vi "weightedPIDs_Controller_CHN.vi"(0 "PID Array":T4(array[cluster])=[{"proportional gain (Kc)"=0.1, "integral time (Ti, min)"=0.1, "derivative time (Td, min)"=0.0}, {"proportional gain (Kc)"=0.1, "integral time (Ti, min)"=0.1, "derivative time (Td, min)"=0.0}, {"proportional gain (Kc)"=0.1, "integral time (Ti, min)"=0.0, "derivative time (Td, min)"=0.0}, {"proportional gain (Kc)"=0.1, "integral time (Ti, min)"=0.0, "derivative time (Td, min)"=0.0}, {"proportional gain (Kc)"=0.37, "integral time (Ti, min)"=0.16, "derivative time (Td, min)"=0.0}, {"proportional gain (Kc)"=0.45, "integral time (Ti, min)"=0.24, "derivative time (Td, min)"=0.0}, {"proportional gain (Kc)"=0.35, "integral time (Ti, min)"=0.133, "derivative time (Td, min)"=0.0}, {"proportional gain (Kc)"=0.25, "integral time (Ti, min)"=0.38, "derivative time (Td, min)"=0.0}], 3 "read.CHN":T6, 4 "calc_CHN":T3, 5 "Parameter_CHN":T2={"alpha_prim_cons"=0.75, "alpha_prim_prod"=0.75, "alpha_sec_cons"=0.25, "alpha_sec_prod"=0.25, "dotQ_norm"=1.0, "T_norm"=3.0, "connection_top"=FALSE, " connection_middle"=FALSE, " connection_bottom"=FALSE}, 6 "FromLogic_CHN":T7={"ControlMode"=enum."weightedPIDs", "CHN_P"=0.0, "S_TM-TG_TH_set"=53.5, "S_TM-HC_TH_set"=50.0, "DeltaT_prim_set"=20.0, "DeltaT_sec_set"=20.0, "A_PU-HC_TH_IMP"=0.0, "A_PU-HC_TH_EXP"=0.0, "A_PU-TG_TH"=0.0, "A_CV-TG_TH"=0.0, "A_PU-HC_TL_IMP"=0.0, "A_PU-HC_TL_EXP"=0.0, "A_PU-TG_TL"=0.0, "A_CV-TG_TL"=0.0, "A_MX-TH"=0.0, "A_PU-TH"=FALSE, "A_PU-TL"=FALSE, "A_BV-HC_TL_IN_open"=FALSE, "A_BV-HC_TL_IN_close"=FALSE, "A_BV-HC_TL_OU_open"=FALSE, "A_BV-HC_TL_OU_close"=FALSE, "A_BV-HC_TH_IN_open"=FALSE, "A_BV-HC_TH_IN_close"=FALSE, "A_BV-HC_TH_OU_open"=FALSE, "A_BV-HC_TH_OU_close"=FALSE, "A_BV-TG_TL_1_open"=FALSE, "A_BV-TG_TL_1_close"=FALSE, "A_BV-TG_TL_2_open"=FALSE, "A_BV-TG_TL_2_close"=FALSE, "A_BV-TG_TL_3_open"=FALSE, "A_BV-TG_TL_3_close"=FALSE, "A_BV-TG_TL_4_open"=FALSE, "A_BV-TG_TL_4_close"=FALSE, "A_BV-TG_TM_1_open"=FALSE, "A_BV-TG_TM_1_close"=FALSE, "A_BV-TG_TM_2_open"=FALSE, "A_BV-TG_TM_2_close"=FALSE, "A_BV-TG_TM_3_open"=FALSE, "A_BV-TG_TM_3_close"=FALSE, "A_BV-TG_TM_4_open"=FALSE, "A_BV-TG_TM_4_close"=FALSE, "A_BV-TG_TH_1_open"=FALSE, "A_BV-TG_TH_1_close"=FALSE, "A_BV-TG_TH_2_open"=FALSE, "A_BV-TG_TH_2_close"=FALSE, "A_BV-TG_TH_3_open"=FALSE, "A_BV-TG_TH_3_close"=FALSE, "A_BV-TG_TH_4_open"=FALSE, "A_BV-TG_TH_4_close"=FALSE}) -> (1 "AO out":T5, 2 "Errorcluster":T1)   [LabVIEW 2018]
uses:
  TypeDef/fromLogic/fromLogic_CHN.ctl
  TypeDef/read/read.CHN.ctl
  TypeDef/Control/CHN/Control_CHN_AO.ctl
  TypeDef/Calc/Calc_CHN.ctl
  TypeDef/Parameters/Parameter_CHN.ctl
  <vilib>/addons/control/pid/pid.llb/PID (DBL).vi
  <vilib>/addons/control/pid/NI_PID_pid.lvlib
panel:
  out "e_pro_sec_Q_is":dbl
  out "e_pro_sec_T_is":dbl
  out "e_pro_sec_T_set":dbl
  out "e_pro_sec_Q_set":dbl
  out "e_pro_prim_Q_is":dbl
  out "e_pro_prim_dT_is":dbl
  out "e_pro_prim_dT_set":dbl
  out "e_pro_prim_Q_set":dbl
  out "e_cons_prim_dT_is":dbl
  out "e_cons_prim_Q_is":dbl
  out "e_cons_prim_dT_set":dbl
  out "e_cons_prim_Q_set":dbl
  out "e_cons_sec_Q_is":dbl
  out "e_cons_sec_dT_is":dbl
  out "e_cons_sec_T_set":dbl
  out "e_cons_sec_Q_set":dbl
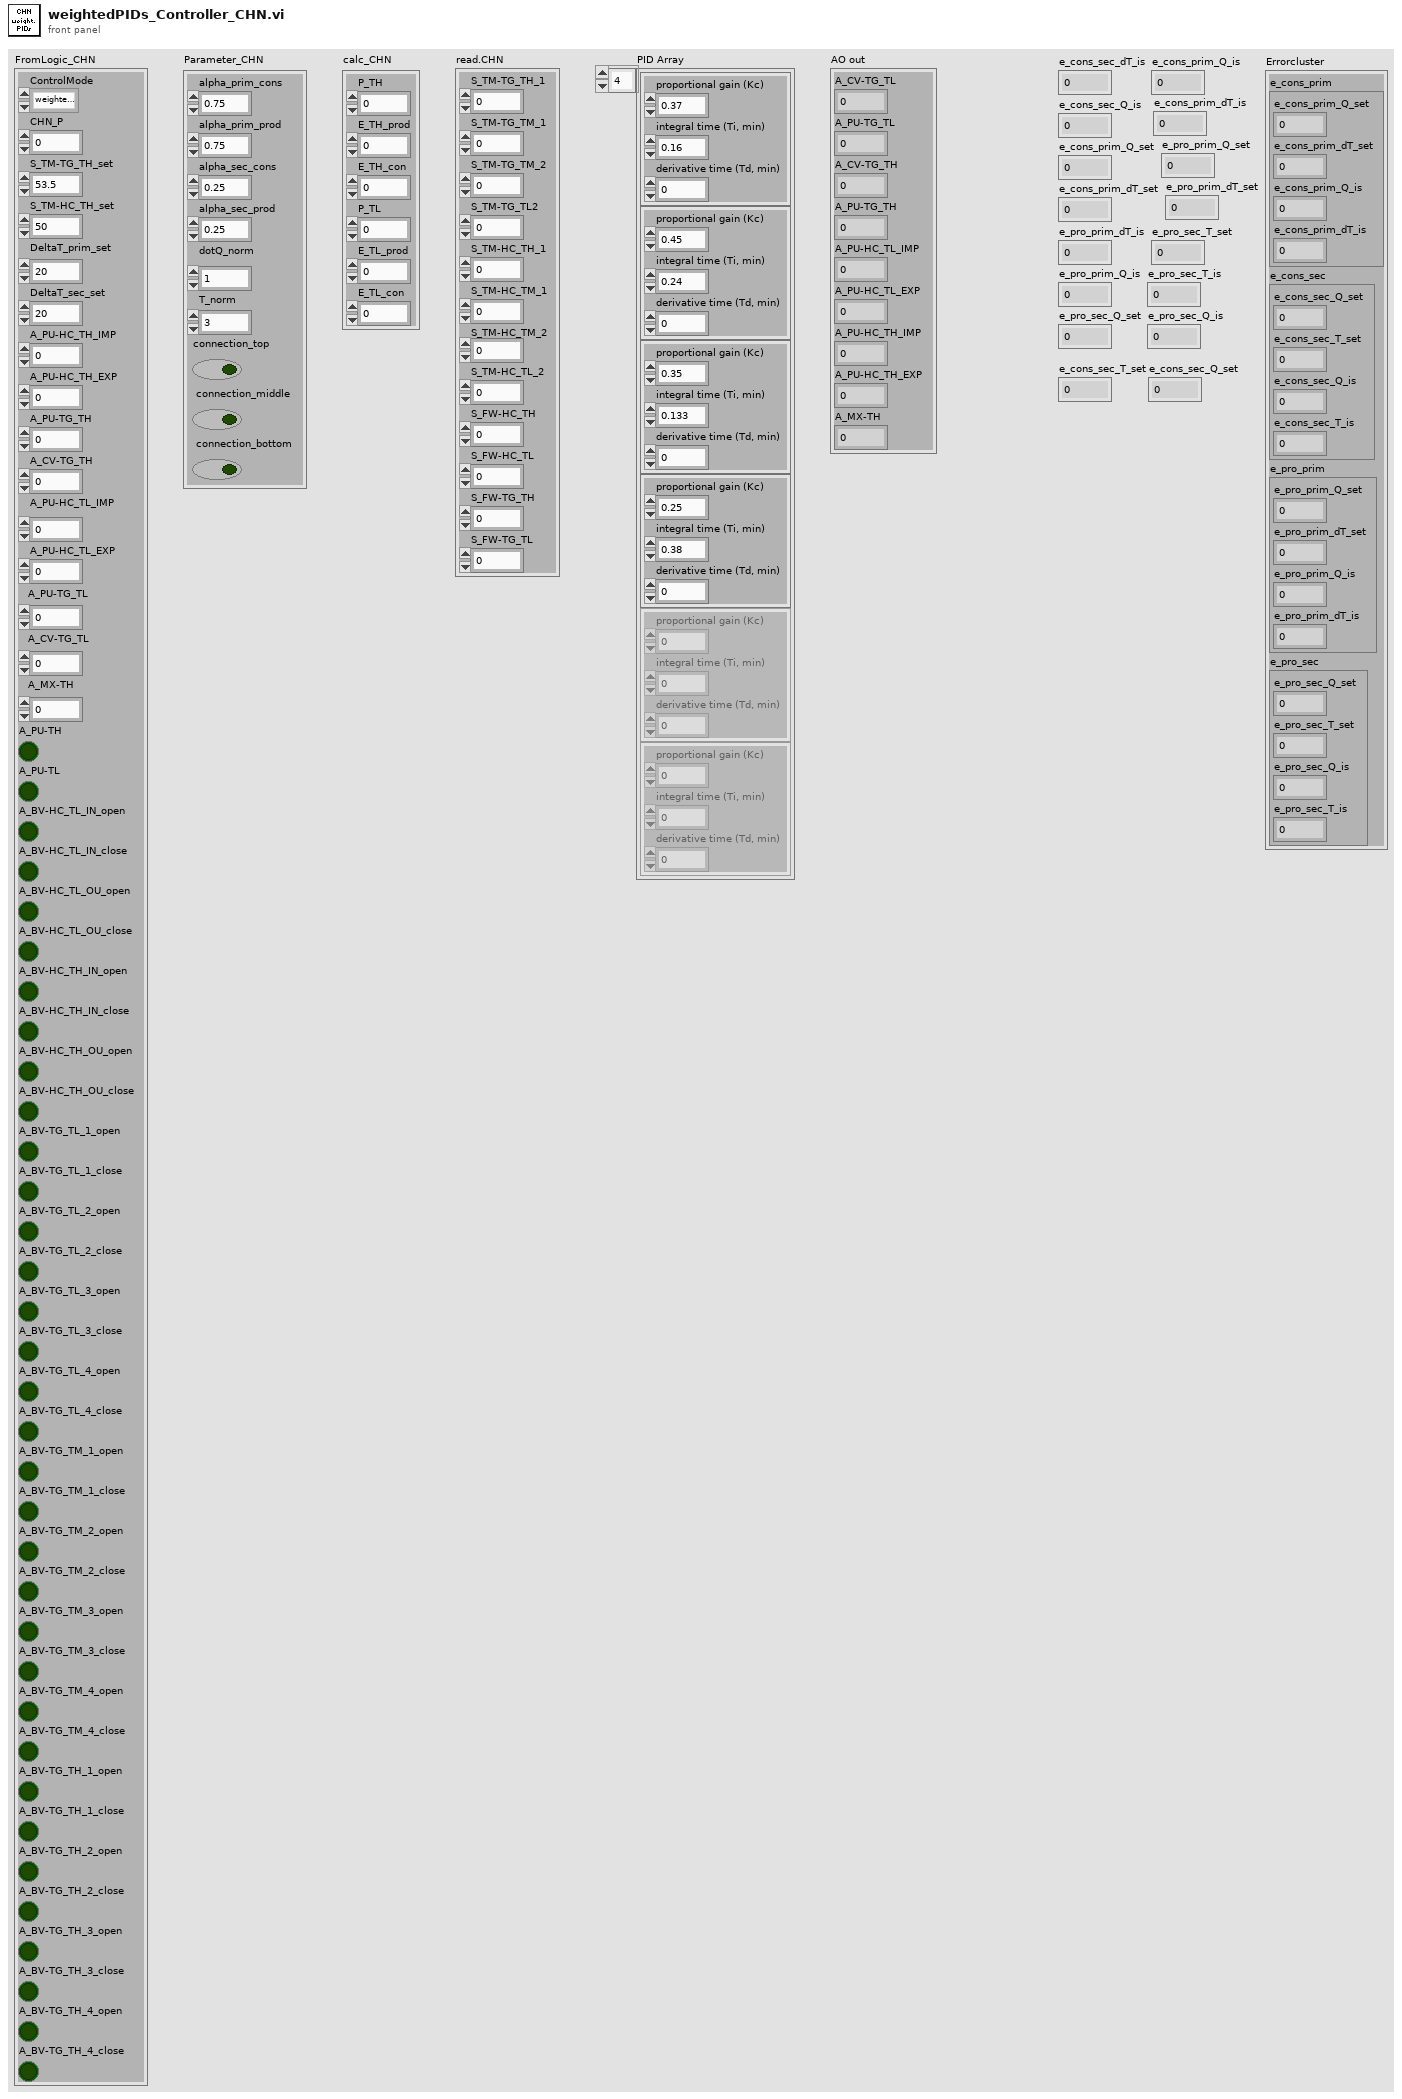
[diagram p1: front panel]
types:
  T1 = cluster{"e_cons_prim":cluster{"e_cons_prim_Q_set ":dbl, "e_cons_prim_dT_set":dbl, "e_cons_prim_Q_is":dbl, "e_cons_prim_dT_is":dbl}, "e_cons_sec":cluster{"e_cons_sec_Q_set ":dbl, "e_cons_sec_T_set":dbl, "e_cons_sec_Q_is":dbl, "e_cons_sec_T_is":dbl}, "e_pro_prim":cluster{"e_pro_prim_Q_set ":dbl, "e_pro_prim_dT_set":dbl, "e_pro_prim_Q_is":dbl, "e_pro_prim_dT_is":dbl}, "e_pro_sec":cluster{"e_pro_sec_Q_set ":dbl, "e_pro_sec_T_set":dbl, "e_pro_sec_Q_is":dbl, "e_pro_sec_T_is":dbl}}
  T2 = typedef "Parameter_CHN.ctl" = cluster{"alpha_prim_cons":dbl, "alpha_prim_prod":dbl, "alpha_sec_cons":dbl, "alpha_sec_prod":dbl, "dotQ_norm":dbl, "T_norm":dbl, "connection_top":bool, " connection_middle":bool, " connection_bottom":bool}
  T3 = typedef "Calc_CHN.ctl" = cluster{"P_TH":dbl, "E_TH_prod":dbl, "E_TH_con":dbl, "P_TL":dbl, "E_TL_prod":dbl, "E_TL_con":dbl}
  T4 = cluster{"proportional gain (Kc)":dbl, "integral time (Ti, min)":dbl, "derivative time (Td, min)":dbl}[]
  T5 = typedef "Control_CHN_AO.ctl" = cluster{"A_CV-TG_TL":dbl, "A_PU-TG_TL":dbl, "A_CV-TG_TH":dbl, "A_PU-TG_TH":dbl, "A_PU-HC_TL_IMP":dbl, "A_PU-HC_TL_EXP":dbl, "A_PU-HC_TH_IMP":dbl, "A_PU-HC_TH_EXP":dbl, "A_MX-TH":dbl}
  T6 = typedef "read.CHN.ctl" = cluster{"S_TM-TG_TH_1":dbl, "S_TM-TG_TM_1":dbl, "S_TM-TG_TM_2":dbl, "S_TM-TG_TL2":dbl, "S_TM-HC_TH_1":dbl, "S_TM-HC_TM_1":dbl, "S_TM-HC_TM_2":dbl, "S_TM-HC_TL_2":dbl, "S_FW-HC_TH":dbl, "S_FW-HC_TL":dbl, "S_FW-TG_TH":dbl, "S_FW-TG_TL":dbl}
  T7 = typedef "fromLogic_CHN.ctl" = cluster{"ControlMode":enum16{"DirectControl", "SimpleController", "weightedPIDs"}, "CHN_P":dbl, "S_TM-TG_TH_set":dbl, "S_TM-HC_TH_set":dbl, "DeltaT_prim_set":dbl, "DeltaT_sec_set":dbl, "A_PU-HC_TH_IMP":dbl, "A_PU-HC_TH_EXP":dbl, "A_PU-TG_TH":dbl, "A_CV-TG_TH":dbl, "A_PU-HC_TL_IMP":dbl, "A_PU-HC_TL_EXP":dbl, "A_PU-TG_TL":dbl, "A_CV-TG_TL":dbl, "A_MX-TH":dbl, "A_PU-TH":bool, "A_PU-TL":bool, "A_BV-HC_TL_IN_open":bool, "A_BV-HC_TL_IN_close":bool, "A_BV-HC_TL_OU_open":bool, "A_BV-HC_TL_OU_close":bool, "A_BV-HC_TH_IN_open":bool, "A_BV-HC_TH_IN_close":bool, "A_BV-HC_TH_OU_open":bool, "A_BV-HC_TH_OU_close":bool, "A_BV-TG_TL_1_open":bool, "A_BV-TG_TL_1_close":bool, "A_BV-TG_TL_2_open":bool, "A_BV-TG_TL_2_close":bool, "A_BV-TG_TL_3_open":bool, "A_BV-TG_TL_3_close":bool, "A_BV-TG_TL_4_open":bool, "A_BV-TG_TL_4_close":bool, "A_BV-TG_TM_1_open":bool, "A_BV-TG_TM_1_close":bool, "A_BV-TG_TM_2_open":bool, "A_BV-TG_TM_2_close":bool, "A_BV-TG_TM_3_open":bool, "A_BV-TG_TM_3_close":bool, "A_BV-TG_TM_4_open":bool, "A_BV-TG_TM_4_close":bool, "A_BV-TG_TH_1_open":bool, "A_BV-TG_TH_1_close":bool, "A_BV-TG_TH_2_open":bool, "A_BV-TG_TH_2_close":bool, "A_BV-TG_TH_3_open":bool, "A_BV-TG_TH_3_close":bool, "A_BV-TG_TH_4_open":bool, "A_BV-TG_TH_4_close":bool}
  T8 = cluster{"e_pro_sec_Q_set ":dbl, "e_pro_sec_T_set":dbl, "e_pro_sec_Q_is":dbl, "e_pro_sec_T_is":dbl}
  T9 = cluster{"e_pro_prim_Q_set ":dbl, "e_pro_prim_dT_set":dbl, "e_pro_prim_Q_is":dbl, "e_pro_prim_dT_is":dbl}
  T10 = cluster{"e_cons_sec_Q_set ":dbl, "e_cons_sec_T_set":dbl, "e_cons_sec_Q_is":dbl, "e_cons_sec_T_is":dbl}
  T11 = cluster{"e_cons_prim_Q_set ":dbl, "e_cons_prim_dT_set":dbl, "e_cons_prim_Q_is":dbl, "e_cons_prim_dT_is":dbl}
  T12 = cluster{"proportional gain (Kc)":dbl, "integral time (Ti, min)":dbl, "derivative time (Td, min)":dbl}
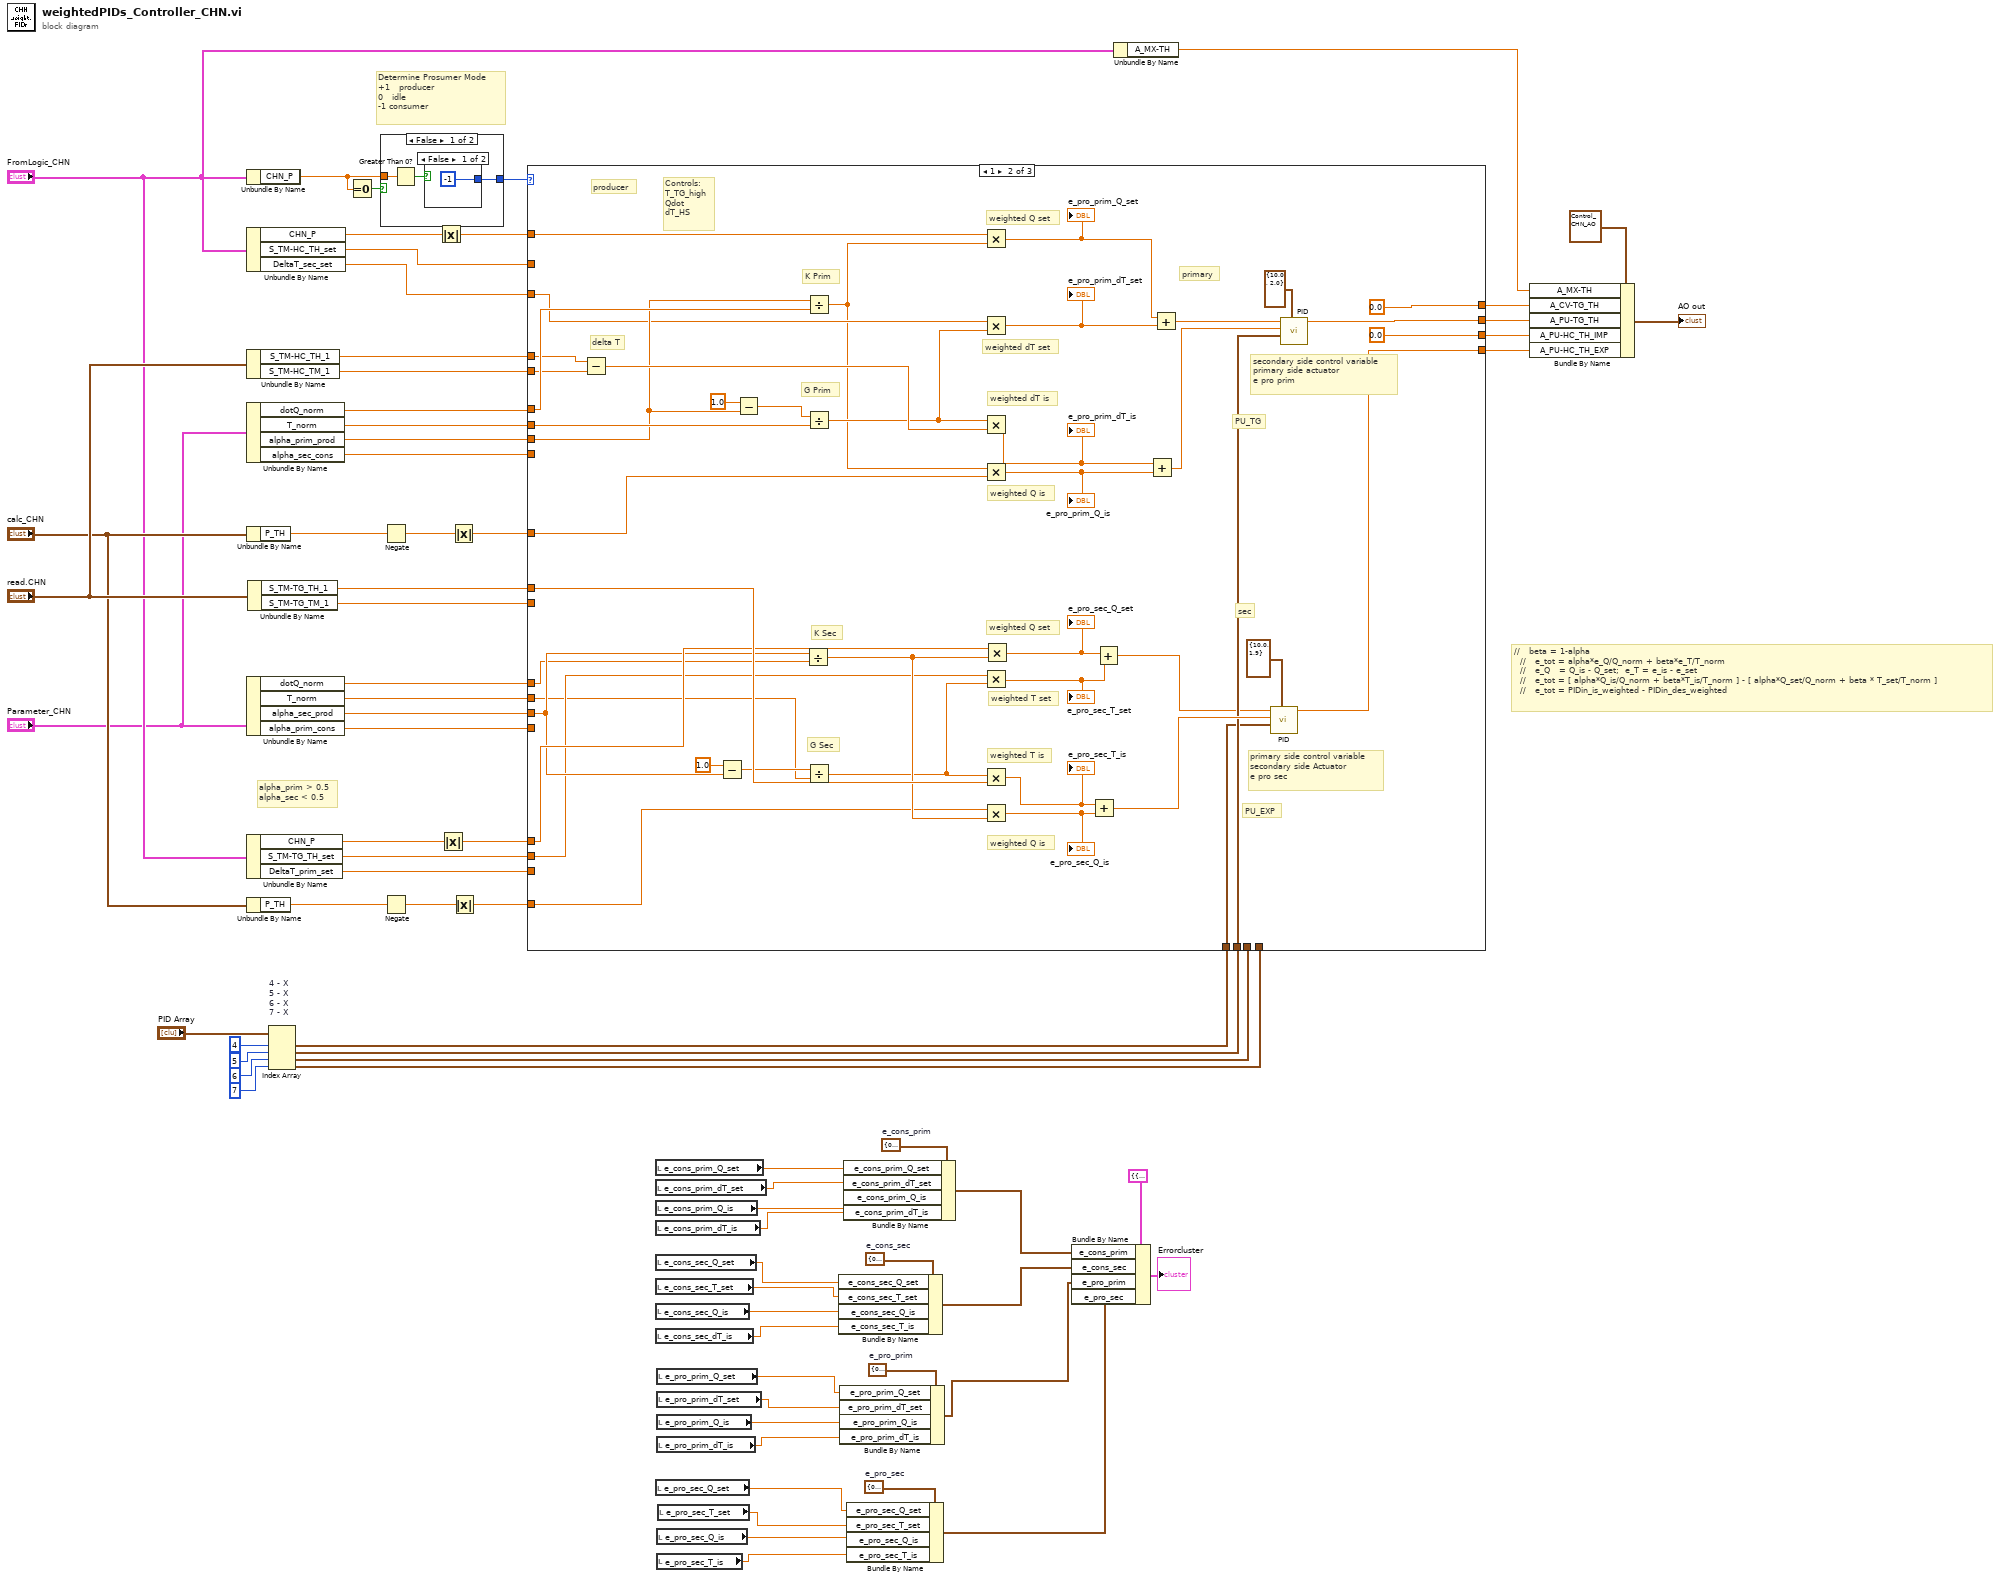
[diagram p0: block diagram]
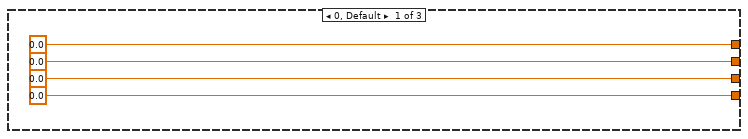
[diagram p2: hidden frame]
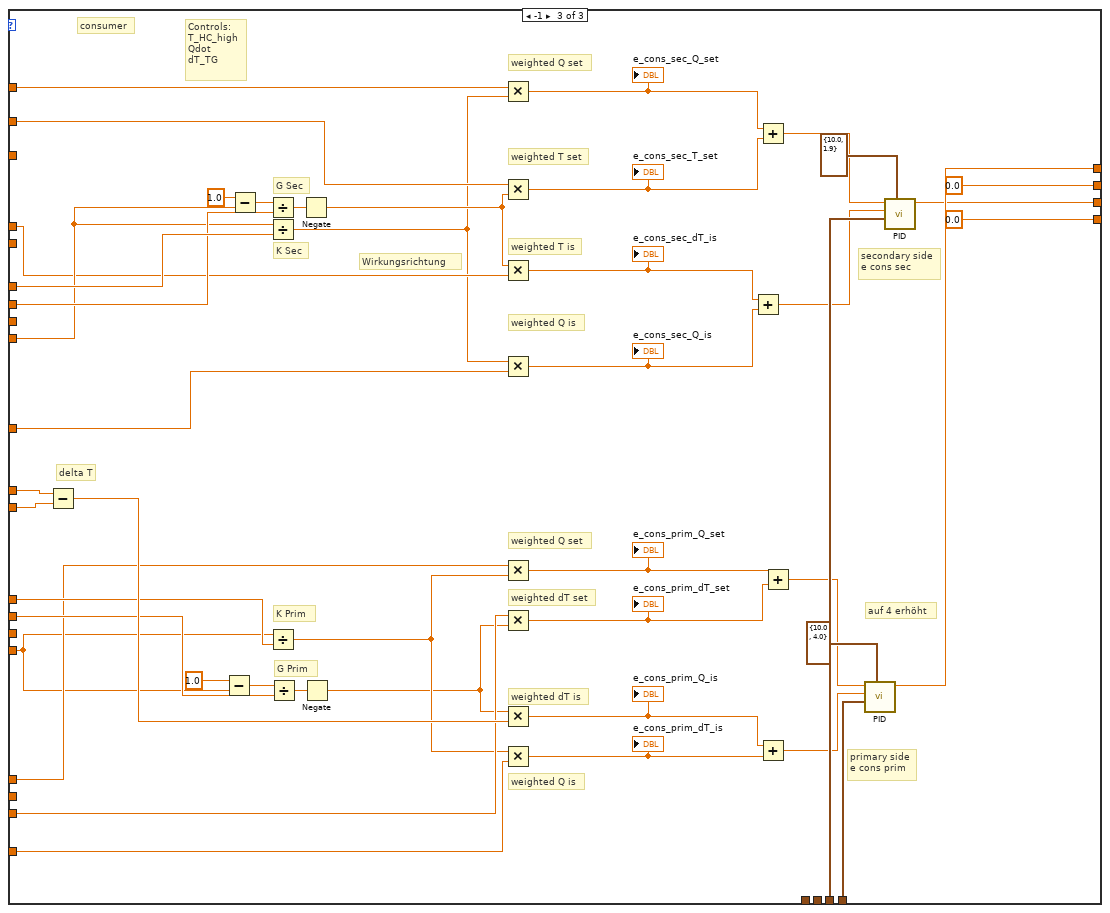
[diagram p3: hidden frame]
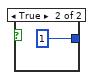
[diagram p4: hidden frame]
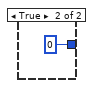
[diagram p5: hidden frame]
diagram:
  w15 = T8 {"e_pro_sec_Q_set "=0.0, "e_pro_sec_T_set"=0.0, "e_pro_sec_Q_is"=0.0, "e_pro_sec_T_is"=0.0}  # e_pro_sec
  w20 = T9 {"e_pro_prim_Q_set "=0.0, "e_pro_prim_dT_set"=0.0, "e_pro_prim_Q_is"=0.0, "e_pro_prim_dT_is"=0.0}  # e_pro_prim
  w25 = T10 {"e_cons_sec_Q_set "=0.0, "e_cons_sec_T_set"=0.0, "e_cons_sec_Q_is"=0.0, "e_cons_sec_T_is"=0.0}  # e_cons_sec
  w26 = T11 {"e_cons_prim_Q_set "=0.0, "e_cons_prim_dT_set"=0.0, "e_cons_prim_Q_is"=0.0, "e_cons_prim_dT_is"=0.0}  # e_cons_prim
  # "alpha_prim > 0.5\nalpha_sec < 0.5"
  # "//   beta = 1-alpha\n  //   e_tot = alpha*e_Q/Q_norm + beta*e_T/T_norm\n  //   e_Q   = Q_is - Q_set;  e_T = e_is - e_set\n  //   e_tot = [ alpha*Q_is/Q_norm + beta*T_is/T_norm ] - [ alpha*Q_set/Q_norm + beta * T_set/T_norm ]\n  //   e_tot = PIDin_is_weighted - PIDin_des_weighted"
  # "Determine Prosumer Mode\n+1   producer\n0   idle\n-1 consumer"
  n1 = Unbundle By Name("FromLogic_CHN") -> ("CHN_P"=w62:dbl)
  n2 = Unbundle By Name("FromLogic_CHN") -> ("CHN_P"=w59:dbl, "S_TM-HC_TH_set"=w58:dbl, "DeltaT_sec_set"=w57:dbl)
  n3 = Unbundle By Name("read.CHN") -> ("S_TM-HC_TH_1"=w36:dbl, "S_TM-HC_TM_1"=w44:dbl)
  n4 = Unbundle By Name("Parameter_CHN") -> ("dotQ_norm"=w43:dbl, "T_norm"=w42:dbl, "alpha_prim_prod"=w37:dbl, "alpha_sec_cons"=w39:dbl)
  n5 = Unbundle By Name("calc_CHN") -> ("P_TH"=w48:dbl)
  n6 = Unbundle By Name("Parameter_CHN") -> ("dotQ_norm"=w55:dbl, "T_norm"=w54:dbl, "alpha_sec_prod"=w61:dbl, "alpha_prim_cons"=w31:dbl)
  n7 = Unbundle By Name("FromLogic_CHN") -> ("CHN_P"=w46:dbl, "S_TM-TG_TH_set"=w38:dbl, "DeltaT_prim_set"=w45:dbl)
  n8 = Unbundle By Name("calc_CHN") -> ("P_TH"=w41:dbl)
  n9 = Unbundle By Name("read.CHN") -> ("S_TM-TG_TH_1"=w56:dbl, "S_TM-TG_TM_1"=w60:dbl)
  n10 = Index Array "4 - X\n5 - X\n6 - X\n7 - X"(array="PID Array", index #1=4 ("index"), index #2=5 ("index"), index #3=6 ("index"), index #4=7 ("index")) -> (element #1=w53:T12, element #2=w52:T12, element #3=w51:T12, element #4=w50:T12)
  n11 = Equal To 0?(x=w62) -> (x = 0?=w68:bool)
  n12 = case shown="False" w68 {
    tunnel: [w76 0] -> w67
    tunnel: w62 -> [w77 _]
    frame False {
      n13 = Greater Than 0?(x=w77) -> (x > 0?=w78:bool)
      n14 = case shown="False" w78 {
        tunnel: [-1 1] -> w76
        frame False {
        }
        frame True {
        }
      }
    }
    frame True {
    }
  }
  n15 = Negate(x=w48) -> (-x=w47:dbl)
  n16 = Negate(x=w41) -> (-x=w40:dbl)
  n17 = Absolute Value(x=w59) -> (abs(x)=w1:dbl)
  n18 = Absolute Value(x=w46) -> (abs(x)=w2:dbl)
  n19 = Absolute Value(x=w47) -> (abs(x)=w4:dbl)
  n20 = Absolute Value(x=w40) -> (abs(x)=w3:dbl)
  n21 = case shown="1" w67 {
    tunnel: [0.0 0.0 w168] -> w66
    tunnel: [0.0 w119 0.0] -> w65
    tunnel: [0.0 0.0 w167] -> w64
    tunnel: [0.0 w120 0.0] -> w63
    tunnel: w61 -> [_ w115 _]
    tunnel: w60 -> [_ _ w170]
    tunnel: w1 -> [_ w95 w153]
    tunnel: w58 -> [_ _ w159]
    tunnel: w57 -> [_ w104 _]
    tunnel: w56 -> [_ w126 w171]
    tunnel: w4 -> [_ w101 w146]
    tunnel: w55 -> [_ w109 w150]
    tunnel: w54 -> [_ w106 w148]
    tunnel: w53 -> [_ w99 _]
    tunnel: w52 -> [_ w100 _]
    tunnel: w51 -> [_ _ w164]
    tunnel: w50 -> [_ _ w163]
    tunnel: w2 -> [_ w118 w141]
    tunnel: w45 -> [_ _ w152]
    tunnel: w44 -> [_ w103 _]
    tunnel: w43 -> [_ w110 w151]
    tunnel: w42 -> [_ w107 w149]
    tunnel: w3 -> [_ w108 w147]
    tunnel: w39 -> [_ _ w145]
    tunnel: w38 -> [_ w111 _]
    tunnel: w37 -> [_ w105 _]
    tunnel: w36 -> [_ w102 w137]
    tunnel: w31 -> [_ _ w140]
    frame 0, Default {
    }
    frame 1 {
      # "delta T"
      # "sec"
      # "K Sec"
      # "G Sec"
      # "primary"
      # "K Prim"
      # "G Prim"
      # "PU_EXP"
      # "PU_TG"
      # "Controls:\nT_TG_high\nQdot\ndT_HS"
      # "producer"
      # "weighted Q is"
      # "weighted T is"
      # "weighted T set"
      # "weighted Q set"
      # "weighted dT is"
      # "weighted Q is"
      # "weighted dT set"
      # "weighted Q set"
      # "secondary side control variable\nprimary side actuator\ne pro prim"
      # "primary side control variable\nsecondary side Actuator\ne pro sec"
      n22 = Subtract(x=w102, y=w103) -> (x-y=w123:dbl)
      n23 = Subtract(x=1.0, y=w115) -> (x-y=w113:dbl)
      n24 = Subtract(x=1.0, y=w105) -> (x-y=w117:dbl)
      n25 = Divide(x=w115, y=w109) -> (x/y=w114:dbl)
      n26 = Divide(x=w105, y=w110) -> (x/y=w94:dbl)
      n27 = Divide(x=w117, y=w107) -> (x/y=w116:dbl)
      n28 = Divide(x=w113, y=w106) -> (x/y=w112:dbl)
      n29 = Multiply(x=w95, y=w94) -> (x*y=w88:dbl)
      "e_pro_prim_Q_set" <- w88
      n30 = Multiply(x=w104, y=w116) -> (x*y=w87:dbl)
      "e_pro_prim_dT_set" <- w87
      n31 = Multiply(x=w116, y=w123) -> (x*y=w93:dbl)
      "e_pro_prim_dT_is" <- w93
      n32 = Multiply(x=w94, y=w101) -> (x*y=w86:dbl)
      "e_pro_prim_Q_is" <- w86
      n33 = Multiply(x=w111, y=w112) -> (x*y=w91:dbl)
      "e_pro_sec_T_set" <- w91
      n34 = Multiply(x=w112, y=w126) -> (x*y=w90:dbl)
      "e_pro_sec_T_is" <- w90
      n35 = Multiply(x=w108, y=w114) -> (x*y=w89:dbl)
      "e_pro_sec_Q_is" <- w89
      n36 = Multiply(x=w118, y=w114) -> (x*y=w92:dbl)
      "e_pro_sec_Q_set" <- w92
      n37 = Add(x=w90, y=w89) -> (x+y=w125:dbl)
      n38 = Add(x=w92, y=w91) -> (x+y=w96:dbl)
      n39 = Add(x=w93, y=w86) -> (x+y=w97:dbl)
      n40 = Add(x=w88, y=w87) -> (x+y=w98:dbl)
      n41 = call-poly <vilib>:"PID.vi"("output range"=cluster{"output high":dbl, "output low":dbl} {"output high"=10.0, "output low"=1.9}, "PID gains"=w99, "process variable"=w125, "setpoint"=w96) -> ("output"=w120:dbl)  [unwired: 6 in, 1 out]
      n42 = call-poly <vilib>:"PID.vi"("output range"=cluster{"output high":dbl, "output low":dbl} {"output high"=10.0, "output low"=2.0}, "PID gains"=w100, "process variable"=w97, "setpoint"=w98) -> ("output"=w119:dbl)  [unwired: 6 in, 1 out]
    }
    frame -1 {
      # "Wirkungsrichtung"
      # "auf 4 erhöht"
      # "K Sec"
      # "G Sec"
      # "K Prim"
      # "G Prim"
      # "delta T"
      # "Controls:\nT_HC_high\nQdot\ndT_TG"
      # "consumer"
      # "weighted Q set"
      # "weighted Q is"
      # "weighted dT is"
      # "weighted dT set"
      # "weighted T is"
      # "weighted T set"
      # "weighted Q is"
      # "weighted Q set"
      # "primary side\ne cons prim"
      # "secondary side\ne cons sec"
      n43 = Subtract(x=w171, y=w170) -> (x-y=w169:dbl)
      n44 = Subtract(x=1.0, y=w140) -> (x-y=w155:dbl)
      n45 = Subtract(x=1.0, y=w145) -> (x-y=w160:dbl)
      n46 = Divide(x=w160, y=w149) -> (x/y=w157:dbl)
      n47 = Divide(x=w145, y=w151) -> (x/y=w136:dbl)
      n48 = Divide(x=w140, y=w150) -> (x/y=w135:dbl)
      n49 = Divide(x=w155, y=w148) -> (x/y=w144:dbl)
      n50 = Negate(x=w157) -> (-x=w142:dbl)
      n51 = Negate(x=w144) -> (-x=w134:dbl)
      n52 = Multiply(x=w153, y=w136) -> (x*y=w162:dbl)
      "e_cons_sec_Q_set" <- w162
      n53 = Multiply(x=w159, y=w142) -> (x*y=w158:dbl)
      "e_cons_sec_T_set" <- w158
      n54 = Multiply(x=w142, y=w137) -> (x*y=w156:dbl)
      "e_cons_sec_dT_is" <- w156
      n55 = Multiply(x=w136, y=w146) -> (x*y=w161:dbl)
      "e_cons_sec_Q_is" <- w161
      n56 = Multiply(x=w141, y=w135) -> (x*y=w139:dbl)
      "e_cons_prim_Q_set" <- w139
      n57 = Multiply(x=w152, y=w134) -> (x*y=w143:dbl)
      "e_cons_prim_dT_set" <- w143
      n58 = Multiply(x=w134, y=w169) -> (x*y=w154:dbl)
      "e_cons_prim_Q_is" <- w154
      n59 = Multiply(x=w135, y=w147) -> (x*y=w138:dbl)
      "e_cons_prim_dT_is" <- w138
      n60 = Add(x=w156, y=w161) -> (x+y=w133:dbl)
      n61 = Add(x=w162, y=w158) -> (x+y=w132:dbl)
      n62 = Add(x=w154, y=w138) -> (x+y=w130:dbl)
      n63 = Add(x=w139, y=w143) -> (x+y=w131:dbl)
      n64 = call-poly <vilib>:"PID.vi"("output range"=cluster{"output high":dbl, "output low":dbl} {"output high"=10.0, "output low"=4.0}, "PID gains"=w163, "process variable"=w130, "setpoint"=w131) -> ("output"=w168:dbl)  [unwired: 6 in, 1 out]
      n65 = call-poly <vilib>:"PID.vi"("output range"=cluster{"output high":dbl, "output low":dbl} {"output high"=10.0, "output low"=1.9}, "PID gains"=w164, "process variable"=w133, "setpoint"=w132) -> ("output"=w167:dbl)  [unwired: 6 in, 1 out]
    }
  }
  n66 = local read "e_cons_prim_Q_set"() -> (w30:dbl)
  n67 = local read "e_cons_prim_dT_set"() -> (w29:dbl)
  n68 = local read "e_cons_prim_Q_is"() -> (w28:dbl)
  n69 = local read "e_cons_prim_dT_is"() -> (w27:dbl)
  n70 = local read "e_cons_sec_Q_set"() -> (w24:dbl)
  n71 = local read "e_cons_sec_T_set"() -> (w23:dbl)
  n72 = local read "e_cons_sec_Q_is"() -> (w22:dbl)
  n73 = local read "e_cons_sec_dT_is"() -> (w21:dbl)
  n74 = local read "e_pro_sec_Q_set"() -> (w14:dbl)
  n75 = local read "e_pro_prim_Q_set"() -> (w19:dbl)
  n76 = local read "e_pro_prim_dT_set"() -> (w18:dbl)
  n77 = local read "e_pro_prim_Q_is"() -> (w17:dbl)
  n78 = local read "e_pro_prim_dT_is"() -> (w16:dbl)
  n79 = local read "e_pro_sec_Q_is"() -> (w12:dbl)
  n80 = local read "e_pro_sec_T_is"() -> (w11:dbl)
  n81 = local read "e_pro_sec_T_set"() -> (w13:dbl)
  n82 = Bundle By Name(cluster=w25, "e_cons_sec_Q_set"=w24, "e_cons_sec_T_set"=w23, "e_cons_sec_Q_is"=w22, "e_cons_sec_T_is"=w21) -> (w8:T10)
  n83 = Bundle By Name(cluster=w20, "e_pro_prim_Q_set"=w19, "e_pro_prim_dT_set"=w18, "e_pro_prim_Q_is"=w17, "e_pro_prim_dT_is"=w16) -> (w7:T9)
  n84 = Bundle By Name(cluster=w26, "e_cons_prim_Q_set"=w30, "e_cons_prim_dT_set"=w29, "e_cons_prim_Q_is"=w28, "e_cons_prim_dT_is"=w27) -> (w9:T11)
  n85 = Bundle By Name(cluster=w15, "e_pro_sec_Q_set"=w14, "e_pro_sec_T_set"=w13, "e_pro_sec_Q_is"=w12, "e_pro_sec_T_is"=w11) -> (w6:T8)
  n86 = Bundle By Name(cluster=T1 {"e_cons_prim"={"e_cons_prim_Q_set "=0.0, "e_cons_prim_dT_set"=0.0, "e_cons_prim_Q_is"=0.0, "e_cons_prim_dT_is"=0.0}, "e_cons_sec"={"e_cons_sec_Q_set "=0.0, "e_cons_sec_T_set"=0.0, "e_cons_sec_Q_is"=0.0, "e_cons_sec_T_is"=0.0}, "e_pro_prim"={"e_pro_prim_Q_set "=0.0, "e_pro_prim_dT_set"=0.0, "e_pro_prim_Q_is"=0.0, "e_pro_prim_dT_is"=0.0}, "e_pro_sec"={"e_pro_sec_Q_set "=0.0, "e_pro_sec_T_set"=0.0, "e_pro_sec_Q_is"=0.0, "e_pro_sec_T_is"=0.0}}, "e_cons_prim"=w9, "e_cons_sec"=w8, "e_pro_prim"=w7, "e_pro_sec"=w6) -> (→"Errorcluster":T1)
  n87 = Unbundle By Name("FromLogic_CHN") -> ("A_MX-TH"=w49:dbl)
  n88 = Bundle By Name(cluster=T5 {"A_CV-TG_TL"=0.0, "A_PU-TG_TL"=0.0, "A_CV-TG_TH"=0.0, "A_PU-TG_TH"=0.0, "A_PU-HC_TL_IMP"=0.0, "A_PU-HC_TL_EXP"=0.0, "A_PU-HC_TH_IMP"=0.0, "A_PU-HC_TH_EXP"=0.0, "A_MX-TH"=0.0} ("AO in"), "A_MX-TH"=w49, "A_CV-TG_TH"=w66, "A_PU-TG_TH"=w65, "A_PU-HC_TH_IMP"=w64, "A_PU-HC_TH_EXP"=w63) -> (→"AO out":T5)
